vi "GetHelp.vi"(11 "RunVIAnalyzer in":refnum<class "RunVIAnalyzer.lvclass">) -> (2 "Help":string, 3 "RunVIAnalyzer out":refnum<class "RunVIAnalyzer.lvclass">)   [LabVIEW 2014, in "RunVIAnalyzer.lvclass"]
uses:
  RunVIAnalyzer.lvclass
panel:
  in  "Help":string="LabVIEWCLI -OperationName RunVIAnalyzer -ConfigPath <path of VI Analyzer configuration file> -ReportPath <Path of VI Analyzer report file> [-ReportSaveType <format of report file>]  [-ConfigPassword <password of config file>] [-ResultsPath <Path of VI Analyzer results file>]\n\n -ConfigPath : Specifies the path to the configuration file (.cfg) that contains VI Analyzer task settings to use in the analysis. You can use a configuration file you saved through the VI Analyzer or the VI Analyzer VIs. Alternatively, you can specify a VI, folder, or LLB to analyze. If you specify an item other than a configuration file, the VI runs all VI Analyzer tests on the specified item.\n -ReportPath : Specifies the path to the report or results file. \n -ReportSaveType : Specifies the format of the report or results file. Use one of the following supported formats:\n      - ASCII: A tab-delimited ASCII file. This is the default.\n      - HTML: An HTML file\n      - \"RSL File\": A VI Analyzer results file. Load this file into the VI Analyzer to view results and address failures. You must enclose this value in quotes. To access the results file on computer other than the one you ran VIAnayzer on, copy the results file to the same relative file location with respect to the source code.\n -ConfigPassword : Specifies the password for the configuration file, if any.\n -ResultsPath : Specifies the path to the results file. If the path is an empty string, LabVIEW ignores the argument."
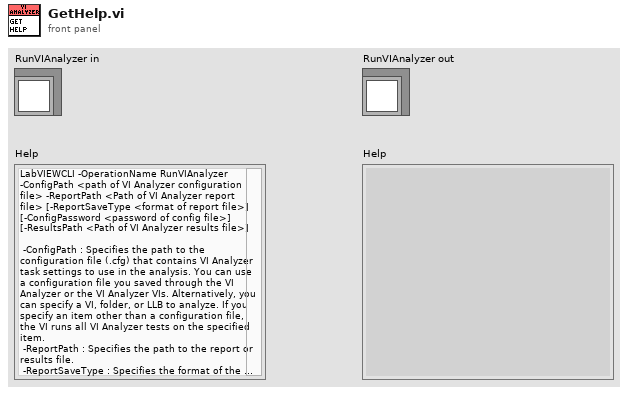
[diagram p1: front panel]
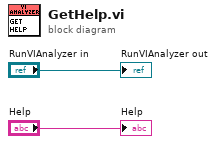
[diagram p0: block diagram]
diagram:
  "RunVIAnalyzer out" <- "RunVIAnalyzer in"
  "Help" <- "Help"
